vi "TxtFile Save_CSM.vi"(8 "error in (no error)":errorcluster, 10 "text":string, 11 "Path":path) -> (0 "error out":errorcluster)   [LabVIEW 2017, in "csm-file-support.lvlib"]
doc: "Write text file."
uses:
  csm-file-support.lvlib
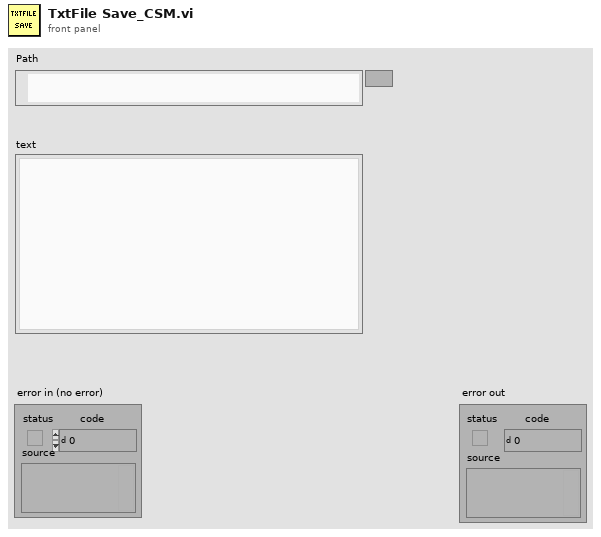
[diagram p1: front panel]
types:
  T1 = enum16{"open", "replace", "create", "open or create", "replace or create", "replace or create with confirmation"}
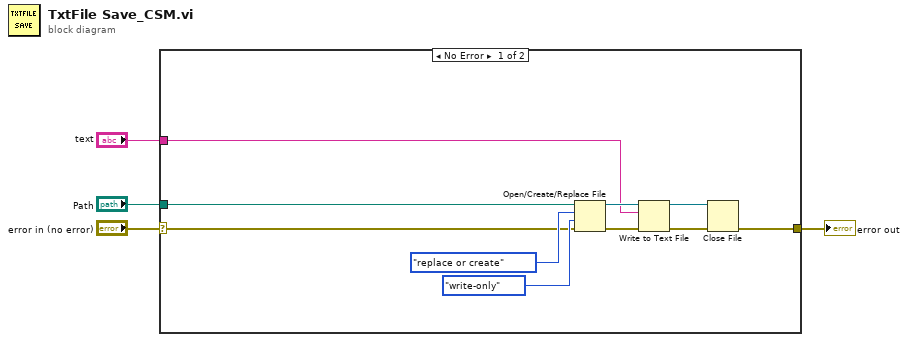
[diagram p0: block diagram]
diagram:
  n1 = case shown="No Error" "error in (no error)" {
    selector: "error in (no error)" -> [w5 w15]
    tunnel: [w8 w15] -> w3
    tunnel: "Path" -> [w6 _]
    tunnel: "text" -> [w7 _]
    frame No Error {
      n2 = Open/Create/Replace File(file path (use dialog)=w6, error in=w5, operation (0:open)=T1."replace or create", access (0:read/write)=enum16{"read/write", "read-only", "write-only"}."write-only") -> (refnum out=w12:refnum<file>, error out=w9:errorcluster)  [unwired: 2 in, 1 out]
      n3 = Write to Text File(file (use dialog)=w12, text=w7, error in=w9) -> (refnum out=w11:refnum<file>, error out=w10:errorcluster)  [unwired: 1 in, 1 out]
      n4 = Close File(refnum=w11, error in=w10) -> (error out=w8:errorcluster)  [unwired: 1 out]
    }
    frame Error {
    }
  }
  "error out" <- w3
